vi "Write Browse Options Prompt.vi"(8 "error in (no error)":errorcluster, 10 "Prompt":string, 11 "Path.lvclass in":refnum<class "Path.lvclass">) -> (0 "error out":errorcluster, 3 "Path.lvclass out":refnum<class "Path.lvclass">)   [LabVIEW 2015, in "Path.lvclass"]
uses:
  Path.lvclass
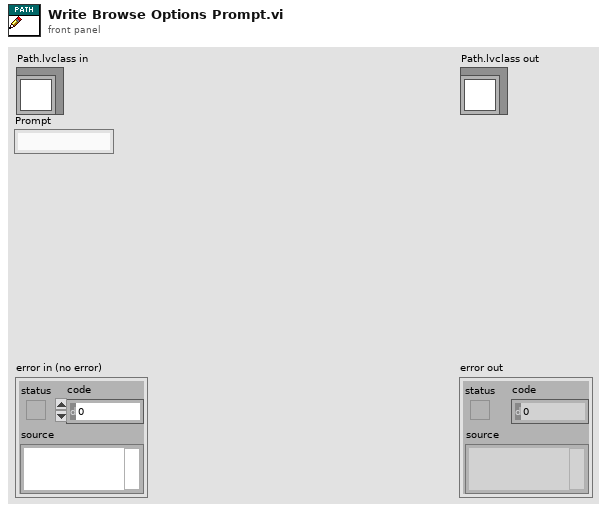
[diagram p1: front panel]
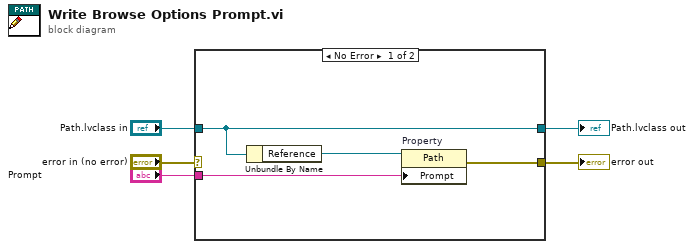
[diagram p0: block diagram]
diagram:
  n1 = case shown="No Error" "error in (no error)" {
    selector: "error in (no error)" -> [_ w11]
    tunnel: [w9 w11] -> w4
    tunnel: [w7 w10] -> w2
    tunnel: "Path.lvclass in" -> [w7 w10]
    tunnel: "Prompt" -> [w8 _]
    frame No Error {
      n2 = Unbundle By Name(w7) -> ("Reference"=w6:refnum<vi>)
      n3 = property on="Property" class="Path"(reference=w6, "Prompt"=w8) -> (error out=w9:errorcluster)  [unwired: 1 in, 1 out]
    }
    frame Error {
    }
  }
  "error out" <- w4
  "Path.lvclass out" <- w2
